vi "VI Statusuebersicht.vi"() -> ()   [LabVIEW 2020, in "Statusuebersicht.lvlib"]
uses:
  Statusuebersicht.lvlib
  Visualisierungs Elemente/String - Ausgabefeld.ctl
  Visualisierungs Elemente/Zahlen-Ausgabefeld.ctl
  FT-IR/FGV FT-IR Gasliste Aktionen.ctl
  Gaszuordnung AO/FGV Gaszuordnung Grenzen&Einheit Aktion.ctl
  Sprachverwaltung/FGV Aktion Tabelle zerlegen.ctl
  FT-IR/FGV FT-IR Diagnose Aktionen.ctl
  FT-IR/FT-IR.lvlib
  cRIO/PC/Kommunikation mit cRIO.lvlib
  Gaszuordnung AO/Gaszuordnung AO.lvlib
  Allgemein/allgemeine Sub-VIs.lvlib
  Sprachverwaltung/Sprachverwaltung.lvlib
  Messdaten/Messdaten.lvlib
panel:
  out "Einheit 2":T1[](array[typedef])
  out "Einheit 1":T1[](array[typedef])
  out "Werte 2":T2[](array[typedef]) format="%.3f"
  out "Werte 1":T2[](array[typedef]) format="%.3f"
  out "Komponenten 2":T1[](array[typedef])
  out "Komponenten 1":T1[](array[typedef])
  # "Statusübersicht"
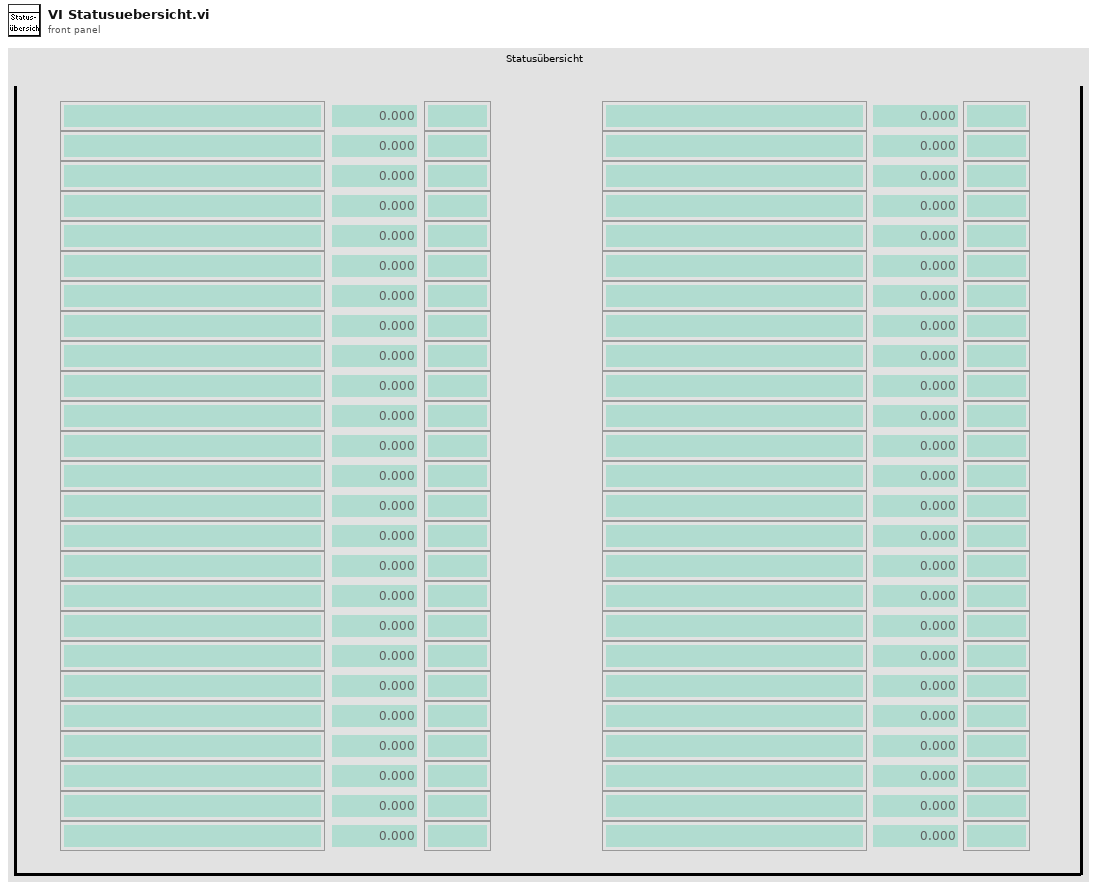
[diagram p1: front panel]
types:
  T1 = typedef "String - Ausgabefeld.ctl" = string
  T2 = typedef "Zahlen-Ausgabefeld.ctl" = sgl
  T3 = typedef "Sprachverwaltung.lvlib/FGV Aktion Tabelle zerlegen.ctl" = enum16{"laden", "vereinzeln", "speichern"}
  T4 = typedef "Gaszuordnung AO.lvlib/FGV Gaszuordnung Grenzen&Einheit Aktion.ctl" = enum16{"Lesen", "Schreiben Min", "Schreiben Max", "Laden", "Speichern"}
  T5 = typedef "FT-IR.lvlib/FGV FT-IR Gasliste Aktionen.ctl" = enum16{"lesen", "Gasliste FT-IR", "Gasliste ausgelesen", "laden", "speichern", "löschen"}
  T6 = typedef "FT-IR.lvlib/FGV FT-IR Diagnose Aktionen.ctl" = enum16{"Lesen", "Diagnose Schreiben", "Min Schreiben", "Max Schreiben"}
  T7 = typedef "FT-IR.lvlib/TOOLweb Interface.lvlib/Typdefinitionen.lvlib/TOOLweb Diagnose.ctl" = cluster{"(14) temperature":sgl, "(15) pressure":sgl, "(16) oxygen":sgl, "(50) diag-igramdc":sgl, "(51) diag-igrampp":sgl, "(52) diag-phaseAngle":sgl, "(53) diag-laserpp":sgl, "(54) diag-laserdc":sgl, "(55) diag-badscan":sgl, "(56) diag-centerburst":sgl, "(57) diag-linearizerCheck":sgl, "(58) diag-SNR":sgl, "(59) diag-sBeamIntensity":sgl}
  T8 = typedef "Verwaltung - cRIO.lvlib/Analog Eingaenge.ctl" = cluster{"AI0: Durchfluss FT-IR":sgl, "AI1: Druck Ausgang":sgl, "AI2: Umgebungsdruck":sgl, "AI3: Druck FT-IR":sgl, "AI4: Druck CalGas":sgl, "AI5: Reserve":sgl, "AI6: Reserve":sgl, "AI7: Reserve":sgl, "Rohwert Durchfluss FT-IR":sgl, "Rohwert Druck Ausgang":sgl, "Rohwert Umgebungsdruck":sgl, "Rohwert Druck FT-IR":sgl, "Rohwert Druck CalGas":sgl, "Rohwert AI5":sgl, "Rohwert AI6":sgl, "Rohwert AI7":sgl, "Rohwert Diffdruck mbar FTIR":sgl}
  T9 = typedef "Verwaltung - cRIO.lvlib/TC Eingaenge.ctl" = cluster{"TC0: Reserve":sgl, "TC1: HL zu FT-IR":sgl, "TC2: HL Extern SP1":sgl, "TC3: HL Extern SP2":sgl, "TC4: Reserve":sgl, "TC5: Reserve":sgl, "TC6: Reserve":sgl, "TC7: Reserve":sgl, "TC8: FT-IR":sgl, "TC9: Reserve":sgl, "TC10: Schaltschrank":sgl, "TC11: Umgebung":sgl}
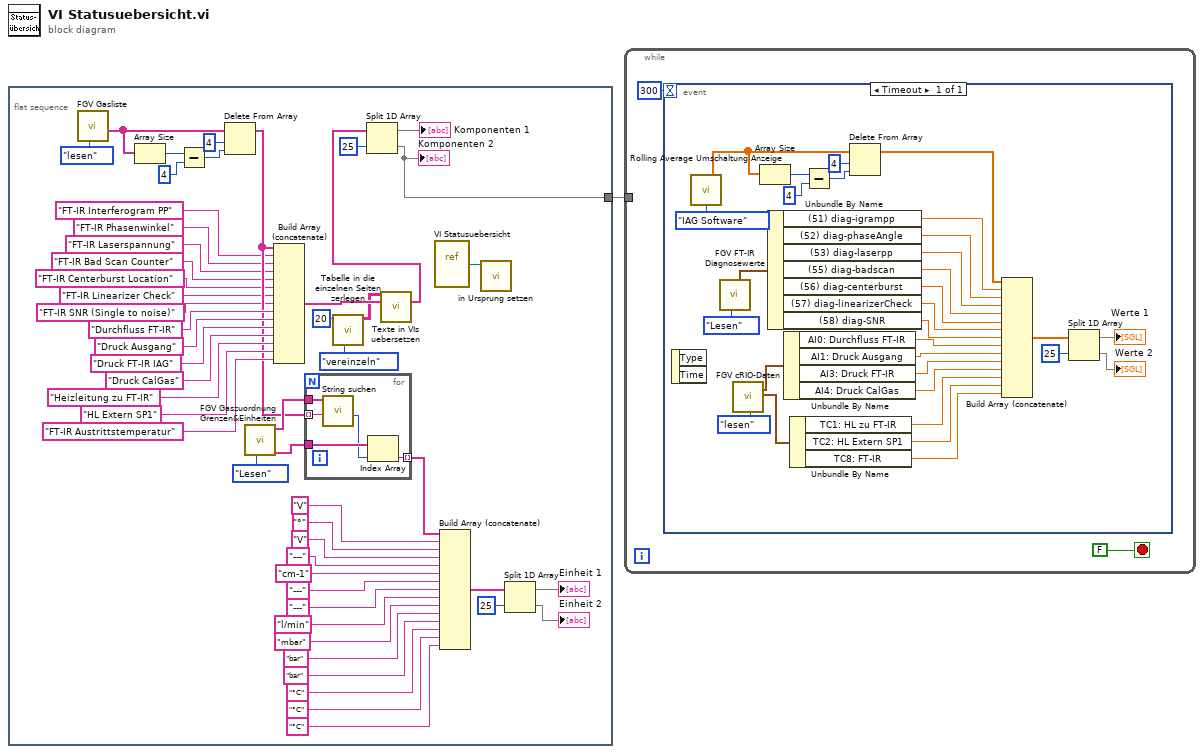
[diagram p0: block diagram]
diagram:
  n1 = flat-sequence {
    tunnel: [w45] -> w1
    frame #0 {
      n2 = call "FGV Gasliste.vi"("Aktionen"=FGV_FT-IR_Gasliste_Aktionen."lesen") -> ("Aktuelle Gasliste gesamt"=w47:T1[])  [unwired: 8 in, 2 out]
      n3 = Array Size(array=w47) -> (size(s)=w52:i32)
      n4 = Subtract(x=w52, y=4) -> (x-y=w50:i32)
      n5 = Delete From Array(array=w47, length=4 ("Länge"), index=w50) -> (array with subset deleted=w23:T1[])  [unwired: 1 out]
      n6 = call "FGV Gaszuordnung Grenzen&Einheiten.vi"("Aktion"=FGV_Gaszuordnung_Grenzen&Einheit_Aktion."Lesen") -> ("Einheit neu"=w36:string[], "Namen neu"=w37:string[])  [unwired: 2 in, 7 out]
      n7 = Build Array (concatenate)(w23, "FT-IR Interferogram PP", "FT-IR Phasenwinkel", "FT-IR Laserspannung", "FT-IR Bad Scan Counter", "FT-IR Centerburst Location", "FT-IR Linearizer Check", "FT-IR SNR (Single to noise)", "Durchfluss FT-IR", "Druck Ausgang", "Druck FT-IR IAG", "Druck CalGas", "Heizleitung zu FT-IR", "HL Extern SP1", "FT-IR Austrittstemperatur") -> (w6:T1[])
      n8 = for {
        tunnel: w37 -> [w56]
        tunnel: w36 -> [w58]
        tunnel: [w57] -> w15 mode=indexing
        tunnel: w23 -> [w54] mode=indexing
        n9 = call "String suchen.vi"("Gasname"=w54, "Such-Namen"=w56) -> ("Index"=w55:i32)  [unwired: 8 in, 1 out]
        n10 = Index Array(array=w58, index=w55) -> (element=w57:string)
      }
      n11 = call "Tabelle in die einzelnen Seiten zerlegen.vi"("Aktion"=FGV_Aktion_Tabelle_zerlegen."vereinzeln", "Index (Seite)"=20) -> ("Sprachliste"=w4:string[][])  [unwired: 7 in, 2 out]
      n12 = call "Texte in VIs uebersetzen.vi"("Sprachliste"=w4, "String-Array zum Übersetzen"=w6) -> ("String-Array zum Übersetzen"=w5:string[])  [unwired: 9 in, 4 out]
      n13 = Split 1D Array(array=w5, index=25 ("Index")) -> (first subarray=→"Komponenten 1":string[], second subarray=w45:string[])
      "Komponenten 2" <- w45
      n14 = vi-ref "VI Statusuebersicht.vi"() -> (w7:refnum<vi>)
      n15 = Build Array (concatenate)(w15, "V", "°", "V", "---", "cm-1", "---", "---", "l/min", "mbar", "bar", "bar", "°C", "°C", "°C") -> (w26:string[])
      n16 = call "in Ursprung setzen.vi"("VI Referenz"=w7) -> ()  [unwired: 10 in, 1 out]
      n17 = Split 1D Array(array=w26, index=25 ("Index")) -> (first subarray=→"Einheit 1":string[], second subarray=→"Einheit 2":string[])
    }
  }
  n18 = while {
    tunnel: w1 -> [_]
    stop <- FALSE stop-if-true
    n19 = event shown="[0] Timeout" {
      selector: _ -> [_]
      dyn-events: _ -> [_]
      timeout: 300 -> [_]
      event Timeout {
        n20 = event-data() -> ()  [unwired: 3 out]
        n21 = call "Rolling Average Umschaltung Anzeige.vi"("Aktion"=enum16{"AK", "IAG Software"}."IAG Software") -> ("Aktuelle Messwerte"=w62:sgl[])  [unwired: 9 in, 5 out]
        n22 = call "FGV FT-IR Diagnosewerte.vi"("Aktionen"=FGV_FT-IR_Diagnose_Aktionen."Lesen") -> ("Diagnose"=w76:T7)  [unwired: 5 in, 5 out]
        n23 = call "FGV cRIO-Daten.vi"("Aktion"=enum16{"lesen", "schreiben"}."lesen") -> ("Analog Input"=w79:T8, "TC Eingänge"=w66:T9)  [unwired: 9 in, 8 out]
        n24 = Array Size(array=w62) -> (size(s)=w88:i32)
        n25 = Unbundle By Name(w76) -> ("(51) diag-igrampp"=w67:sgl, "(52) diag-phaseAngle"=w68:sgl, "(53) diag-laserpp"=w69:sgl, "(55) diag-badscan"=w70:sgl, "(56) diag-centerburst"=w71:sgl, "(57) diag-linearizerCheck"=w72:sgl, "(58) diag-SNR"=w73:sgl)
        n26 = Unbundle By Name(w79) -> ("AI0: Durchfluss FT-IR"=w80:sgl, "AI1: Druck Ausgang"=w81:sgl, "AI3: Druck FT-IR"=w82:sgl, "AI4: Druck CalGas"=w83:sgl)
        n27 = Unbundle By Name(w66) -> ("TC1: HL zu FT-IR"=w65:sgl, "TC2: HL Extern SP1"=w64:sgl, "TC8: FT-IR"=w63:sgl)
        n28 = Subtract(x=w88, y=4) -> (x-y=w86:i32)
        n29 = Delete From Array(array=w62, length=4 ("Länge"), index=w86) -> (array with subset deleted=w74:sgl[])  [unwired: 1 out]
        n30 = Build Array (concatenate)(w74, w67, w68, w69, w70, w71, w72, w73, w80, w81, w82, w83, w65, w64, w63) -> (w77:sgl[])
        n31 = Split 1D Array(array=w77, index=25 ("Index")) -> (first subarray=→"Werte 1":sgl[], second subarray=→"Werte 2":sgl[])
      }
    }
  }
